vi "Association Add.vi"(8 "error in (no error)":errorcluster, 9 "iInstrument (0)":i32, 10 "iStation (0)":i32, 11 "Connection Refnum":T1) -> (0 "error out":errorcluster, 3 "Connection Refnum":T1)   [LabVIEW 2011]
uses:
  SI.LIB/ODBC/SQL Controls/Connection Refnum.ctl
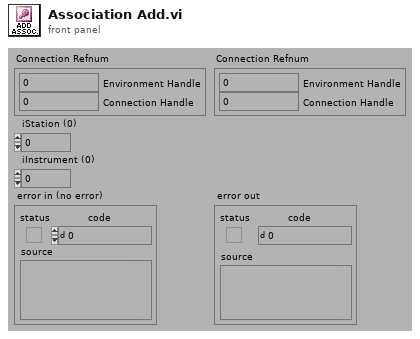
[diagram p1: front panel]
types:
  T1 = typedef "Connection Refnum.ctl" = cluster{"Environment Handle":i32, "Connection Handle":i32}
  T2 = typedef "Statement Refnum.ctl" = cluster{"Statement Handle":i32, "Parameter Number":u16}
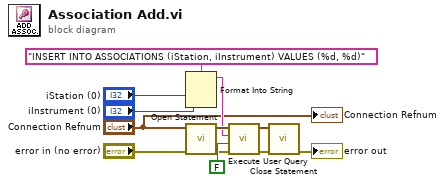
[diagram p0: block diagram]
diagram:
  n1 = Format Into String(format string="INSERT INTO ASSOCIATIONS (iStation, iInstrument) VALUES (%d, %d)" ("User Query"), "iStation (0)", "iInstrument (0)") -> (resulting string=w6:string)  [unwired: 2 in, 1 out]
  n2 = call "Open Statement.vi"("error in (no error)"="error in (no error)", "Connection Refnum"="Connection Refnum") -> ("error out"=w9:errorcluster, "Statement Refnum"=w8:T2)  [unwired: 4 out]
  n3 = call "Execute User Query.vi"("error in (no error)"=w9, "Return Data? (f)"=FALSE, "User Query"=w6, "Statement Refnum"=w8) -> ("error out"=w10:errorcluster, "Statement Refnum"=w11:T2)  [unwired: 2 out]
  n4 = call "Close Statement.vi"("error in (no error)"=w10, "Statement Refnum"=w11) -> ("error out"=→"error out":errorcluster)  [unwired: 5 out]
  "Connection Refnum" <- "Connection Refnum"
